vi "Roots_Function.vi"() -> ()   [LabVIEW 2019]
uses:
  <vilib>/Analysis/polynomials.llb/Polynomial Roots (DBL).vi
  <vilib>/Analysis/NI_AALPro.lvlib
panel:
  out "Roots 3":dbl[](array[numeric])
  in  "Poly(C->B->A)":dbl[](array[numeric])
  in  "Poly":bool
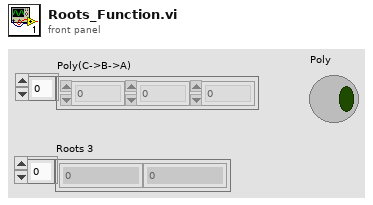
[diagram p1: front panel]
types:
  T1 = cluster{"Poly(C->B->A)[0]":dbl, "Poly(C->B->A)[1]":dbl, "Poly(C->B->A)[2]":dbl, "Poly(C->B->A)[3]":dbl, "Poly(C->B->A)[4]":dbl, "Poly(C->B->A)[5]":dbl, "Poly(C->B->A)[6]":dbl, "Poly(C->B->A)[7]":dbl, "Poly(C->B->A)[8]":dbl}
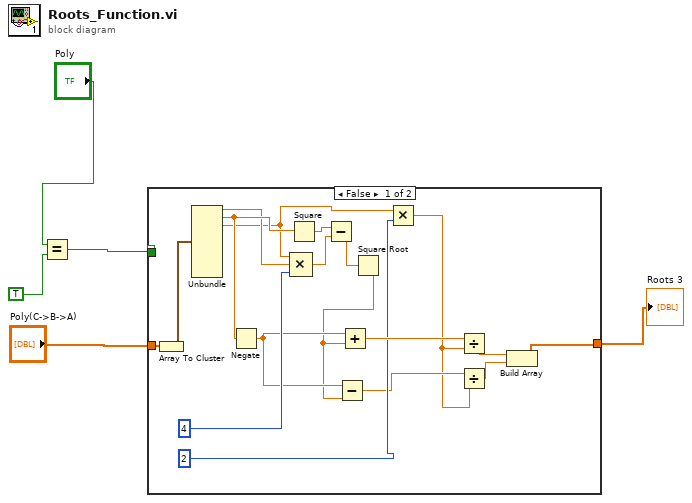
[diagram p0: block diagram]
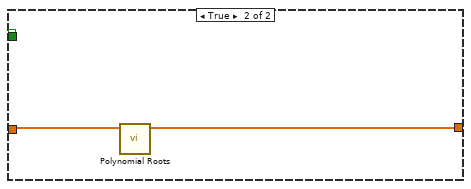
[diagram p2: hidden frame]
diagram:
  n1 = Equal?(x="Poly", y=TRUE) -> (x = y?=w3:bool)
  n2 = case shown="False" w3 {
    selector: w3 -> [_ w26]
    tunnel: [_ w26] -> _
    tunnel: "Poly(C->B->A)" -> [w23 w24]
    tunnel: [w15 w25] -> w1
    frame False {
      n3 = Array To Cluster(array=w23) -> (cluster=w22:T1)
      n4 = Unbundle(w22) -> ("Poly(C->B->A)[0]"=w12:dbl, "Poly(C->B->A)[1]"=w20:dbl, "Poly(C->B->A)[2]"=w11:dbl)  [unwired: 6 out]
      n5 = Negate(x=w20) -> (-x=w7:dbl)
      n6 = Square(x=w20) -> (x^2=w10:dbl)
      n7 = Compound Arithmetic op=MULTIPLY(w11, w12, 4) -> (w9:dbl)
      n8 = Subtract(x=w10, y=w9) -> (x-y=w8:dbl)
      n9 = Square Root(x=w8) -> (sqrt(x)=w6:dbl)
      n10 = Subtract(x=w7, y=w6) -> (x-y=w17:dbl)
      n11 = Add(x=w7, y=w6) -> (x+y=w19:dbl)
      n12 = Multiply(x=w11, y=2) -> (x*y=w16:dbl)
      n13 = Divide(x=w19, y=w16) -> (x/y=w14:dbl)
      n14 = Divide(x=w17, y=w16) -> (x/y=w13:dbl)
      n15 = Build Array(w14, w13) -> (w15:dbl[])
    }
    frame True {
      n16 = call-poly <vilib>:"Polynomial Roots.vi"("P(x)"=w24) -> ("Roots"=w25:cdb[])  [unwired: 9 in, 1 out]
    }
  }
  "Roots 3" <- w1
